vi "创建波形.vi"() -> ()   [LabVIEW 2010]
uses:
  <vilib>/Analysis/NI_AALBase.lvlib
panel:
  out "输出波形":waveform(dbl)
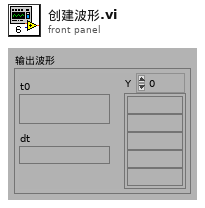
[diagram p1: front panel]
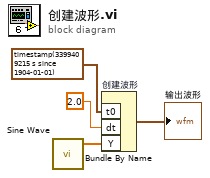
[diagram p0: block diagram]
diagram:
  n1 = call <vilib>:"Sine Wave.vi"() -> ("sine wave"=w4:dbl[])  [unwired: 5 in, 2 out]
  n2 = Bundle By Name "创建波形"("t0"=timestamp(3399409215 s since 1904-01-01), "dt"=2.0, "Y"=w4) -> (→"输出波形":waveform(dbl))  [unwired: 1 in]
